vi "error test.vi"() -> ()   [LabVIEW 2012]
uses:
  SDL.dll
panel:
  out "return type 2":string
  out "return type":string
  out "error out":errorcluster
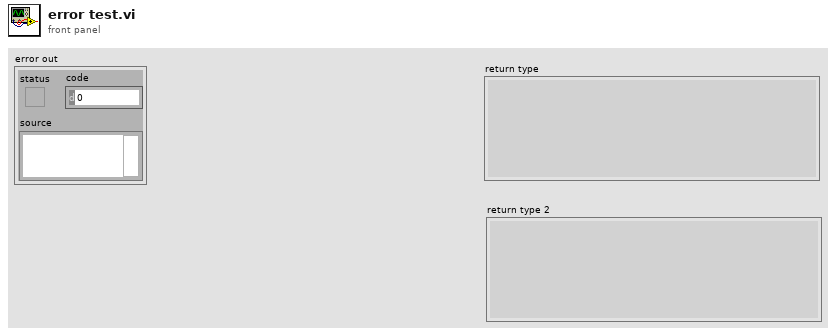
[diagram p1: front panel]
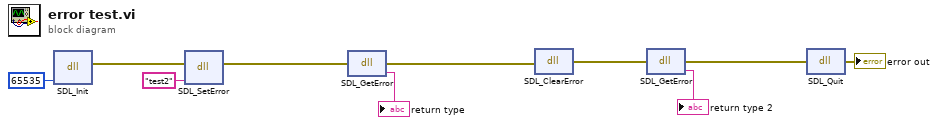
[diagram p0: block diagram]
diagram:
  n1 = dll-call lib="C:/dev/SDL/LabVIEW/libSDL/SDL.dll" fn="SDL_Init"("flags"=u32 65535) -> (error out=w7:errorcluster)  [unwired: 5 in, 1 out]
  n2 = dll-call lib="C:/dev/SDL/LabVIEW/libSDL/SDL.dll" fn="SDL_SetError"(error in=w7, "fmt"="test2") -> (error out=w5:errorcluster)  [unwired: 4 in, 1 out]
  n3 = dll-call lib="C:/dev/SDL/LabVIEW/libSDL/SDL.dll" fn="SDL_GetError"(error in=w5) -> (error out=w4:errorcluster, "return type"=→"return type":string)  [unwired: 2 in, 1 out]
  n4 = dll-call lib="C:/dev/SDL/LabVIEW/libSDL/SDL.dll" fn="SDL_ClearError"(error in=w4) -> (error out=w2:errorcluster)  [unwired: 3 in, 1 out]
  n5 = dll-call lib="C:/dev/SDL/LabVIEW/libSDL/SDL.dll" fn="SDL_GetError"(error in=w2) -> (error out=w1:errorcluster, "return type"=→"return type 2":string)  [unwired: 2 in, 1 out]
  n6 = dll-call lib="C:/dev/SDL/LabVIEW/libSDL/SDL.dll" fn="SDL_Quit"(error in=w1) -> (error out=→"error out":errorcluster)  [unwired: 3 in, 1 out]
